vi "Revision Query.vi"(8 "error in (no error)":errorcluster, 10 "Node (3)":u8=3 caption="Node" min=3 max=128 step=1, 11 "VISA resource name":refnum<visa-resource-name>) -> (0 "error out":errorcluster, 1 "Instrument Firmware Revision":string, 2 "Instrument Driver Revision":string, 3 "VISA resource name out":refnum<visa-resource-name>, 4 "Instrument Modelnumber":string)   [LabVIEW 2024, in "Bronkhorst FLOW-BUS.lvlib"]
doc: "Queries the current instrument firmware revision, instrument driver revision, and the instruments model number.\nRefer to the Readme file for detailed driver information including modification history."
uses:
  Bronkhorst FLOW-BUS.lvlib
  Private/FLOW-BUS RW.ctl
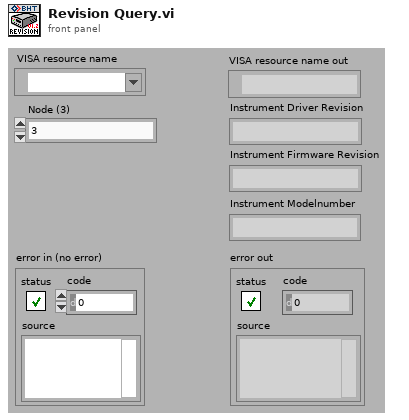
[diagram p1: front panel]
types:
  T1 = typedef "Bronkhorst FLOW-BUS.lvlib/FLOW-BUS RW.ctl" = cluster{"Node Address (3)":u8, "Communication Command":enum16{"Status message", "Send parameter with destination address and 00 response", "Send parameter with destination address", "Request parameter"}, "Process (0)":u16, "Parameter (0)":u16, "Data Type (0: Character)":enum16{"Character", "Integer", "Float or Long", "String"}, "Data for Char or Int (0)":u32, "Data for Float or Long (0)":sgl, "Data for String":string, "Length of Requested String (0)":u8}
  T2 = enum32{"invalid app kind", "Development System", "Run Time System", "Student Edition", "Embedded LabVIEW", "Evaluation", "Custom"}
  T3 = cluster{"Major":u16, "Minor":u16, "Fix":u16, "Build":u16}
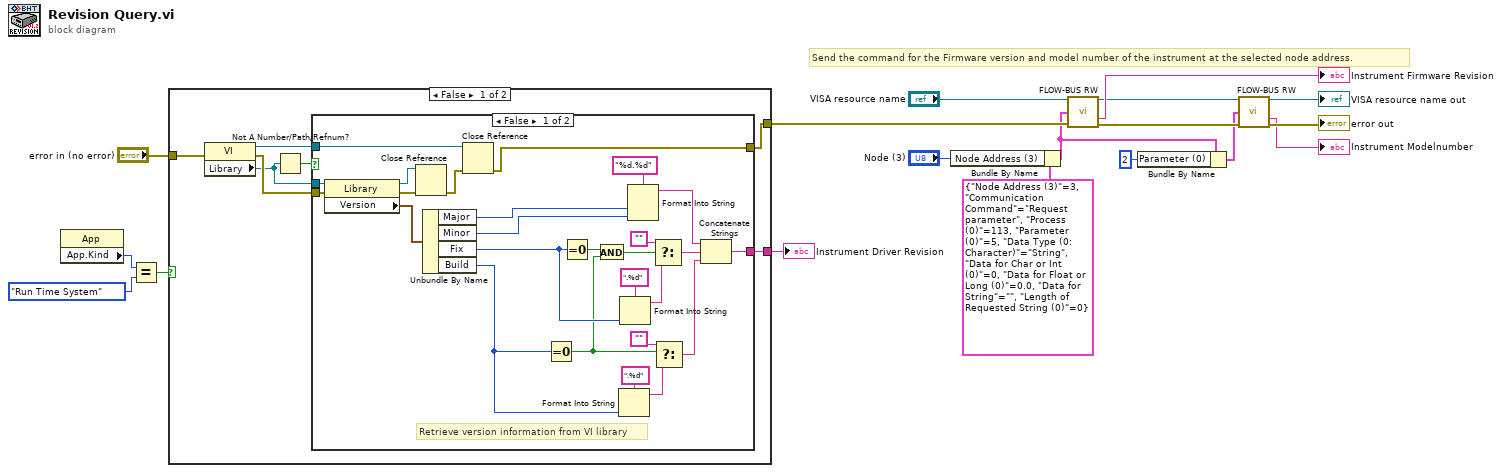
[diagram p0: block diagram]
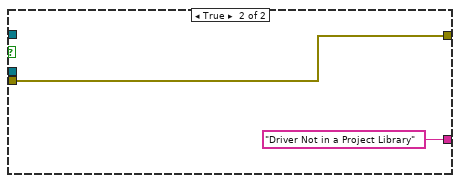
[diagram p2: hidden frame]
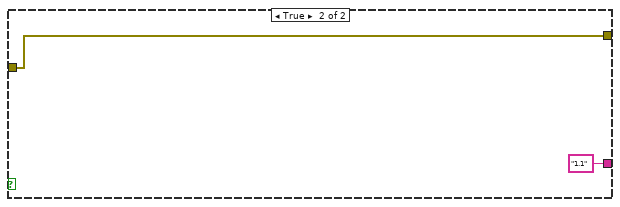
[diagram p3: hidden frame]
diagram:
  # "Send the command for the Firmware version and model number of the instrument at the selected node address."
  n1 = property class="App"() -> ("App.Kind"=w15:T2)  [unwired: 2 in, 2 out]
  n2 = Equal?(x=w15, y=T2."Run Time System" ("Application:Kind")) -> (x = y?=w16:bool)
  n3 = case shown="False" w16 {
    tunnel: [w21 "1.1"] -> w18
    tunnel: "error in (no error)" -> [w20 w54]
    tunnel: [w19 w54] -> w12
    frame False {
      n4 = property class="VI"(error in=w20) -> (reference out=w25:refnum<vi>, error out=w24:errorcluster, "Library"=w23:refnum<vi>)  [unwired: 1 in]
      n5 = Not A Number/Path/Refnum?(number/path/refnum=w23) -> (NaN/Path/Refnum?=w22:bool)
      n6 = case shown="False" w22 {
        tunnel: w25 -> [w48 _]
        tunnel: w24 -> [w33 w53]
        tunnel: [w28 w53] -> w19
        tunnel: [w27 "Driver Not in a Project Library"] -> w21
        tunnel: w23 -> [w26 _]
        frame False {
          # "Retrieve version information from VI library"
          n7 = property class="Library"(reference=w26, error in=w33) -> (reference out=w50:refnum<vi>, error out=w51:errorcluster, "Version"=w47:T3)
          n8 = Close Reference(reference=w50, error in (no error)=w51) -> (error out=w49:errorcluster)
          n9 = Unbundle By Name(w47) -> ("Major"=w36:u16, "Minor"=w35:u16, "Fix"=w32:u16, "Build"=w34:u16)
          n10 = Close Reference(reference=w48, error in (no error)=w49) -> (error out=w28:errorcluster)
          n11 = Equal To 0?(x=w34) -> (x = 0?=w30:bool)
          n12 = Equal To 0?(x=w32) -> (x = 0?=w31:bool)
          n13 = And(x=w31, y=w30) -> (x .and. y?=w29:bool)
          n14 = Format Into String(format string=".%d", w34) -> (resulting string=w40:string)  [unwired: 2 in, 1 out]
          n15 = Format Into String(format string=".%d", w32) -> (resulting string=w44:string)  [unwired: 2 in, 1 out]
          n16 = Format Into String(format string="%d.%d", w36, w35) -> (resulting string=w42:string)  [unwired: 2 in, 1 out]
          n17 = Select(t="", s=w29, f=w44) -> (s? t:f=w41:string)
          n18 = Select(t="", s=w30, f=w40) -> (s? t:f=w37:string)
          n19 = Concatenate Strings(w42, w41, w37) -> (w27:string)
        }
        frame True {
        }
      }
    }
    frame True {
    }
  }
  "Instrument Driver Revision" <- w18
  n20 = Bundle By Name(cluster=T1 {"Node Address (3)"=3, "Communication Command"=enum."Request parameter", "Process (0)"=113, "Parameter (0)"=5, "Data Type (0: Character)"=enum."String", "Data for Char or Int (0)"=0, "Data for Float or Long (0)"=0.0, "Data for String"="", "Length of Requested String (0)"=0} ("FLOW-BUS Command Settings"), "Node Address (3)"="Node (3)") -> (w5:T1)
  n21 = call "FLOW-BUS RW.vi"("VISA resource name"="VISA resource name", "FLOW-BUS Command Settings"=w5, "error in (no error)"=w12) -> ("VISA resource name out"=w8:refnum<visa-resource-name>, "Requested String"=→"Instrument Firmware Revision":string, "error out"=w7:errorcluster)  [unwired: 8 in, 2 out]
  n22 = Bundle By Name(cluster=w5, "Parameter (0)"=u16 2) -> (w6:T1)
  n23 = call "FLOW-BUS RW.vi"("VISA resource name"=w8, "FLOW-BUS Command Settings"=w6, "error in (no error)"=w7) -> ("VISA resource name out"=→"VISA resource name out":refnum<visa-resource-name>, "Requested String"=→"Instrument Modelnumber":string, "error out"=→"error out":errorcluster)  [unwired: 8 in, 2 out]
